vi "Add Item.vi"(6 "ForceAdd(F)":bool, 7 "Type":refnum<class "Generic.lvclass">, 8 "错误输入（无错误）":errorcluster, 9 "TypeGUID":string, 10 "Name":string, 11 "Section in":refnum<data-value>) -> (0 "错误输出":errorcluster, 2 "Item":refnum<data-value>, 3 "Section out":refnum<data-value>, 4 "Newly Created?":bool)   [LabVIEW 2013, in "Hierarchy Framework.lvlib" / "Section.lvclass"]
uses:
  Section.lvclass
  Item/Item.lvclass
  Generic/Generic.lvclass
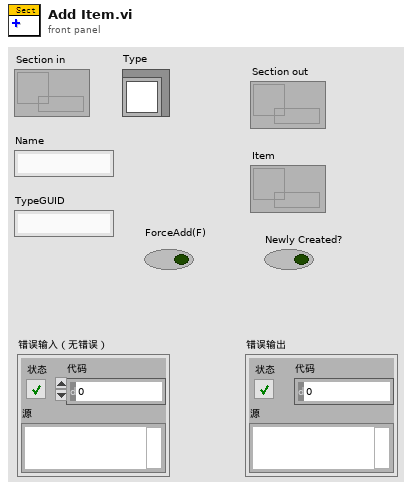
[diagram p1: front panel]
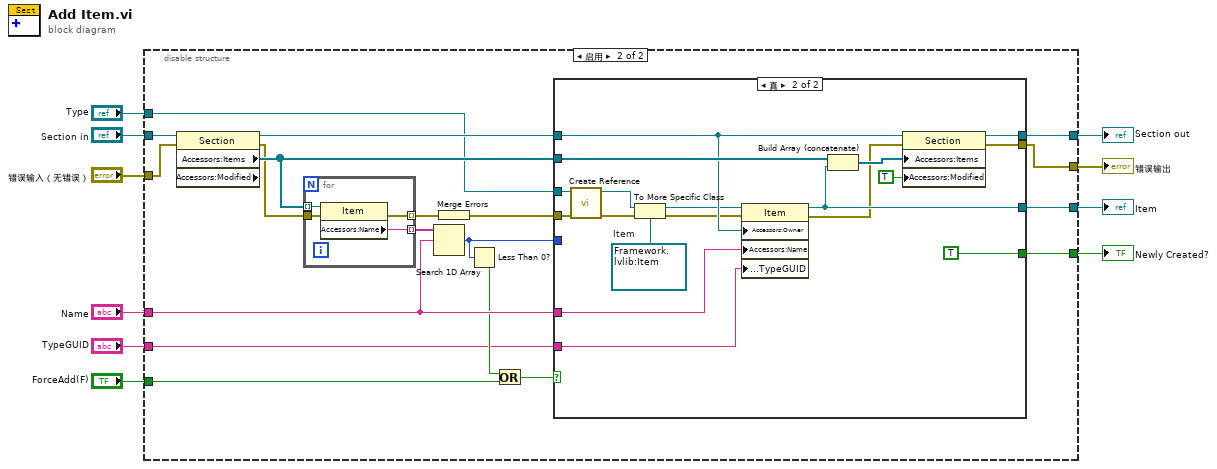
[diagram p0: block diagram]
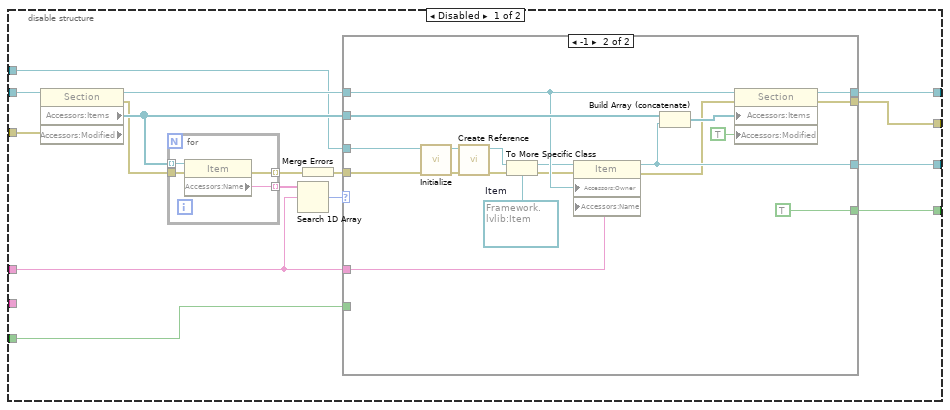
[diagram p2: hidden frame]
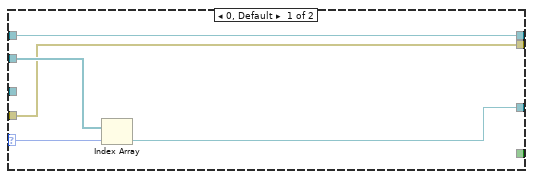
[diagram p3: hidden frame]
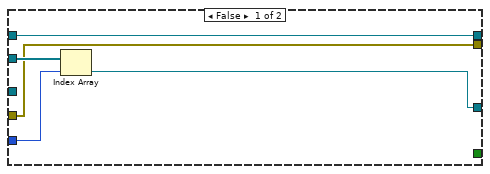
[diagram p4: hidden frame]
diagram:
  n1 = disable-structure shown="启用" {
    disable-tunnel: [w25 w72] -> w10
    disable-tunnel: [w24 w71] -> w9
    disable-tunnel: "Section in" -> [w23 w70]
    disable-tunnel: "错误输入（无错误）" -> [w22 w69]
    disable-tunnel: [w21 w68] -> w6
    disable-tunnel: "Name" -> [w20 w67]
    disable-tunnel: [w13 w61] -> w4
    disable-tunnel: "ForceAdd(F)" -> [w12 w58]
    disable-tunnel: "Type" -> [w11 w60]
    disable-tunnel: "TypeGUID" -> [_ w55]
    frame Disabled {
      n2 = property class="Section" props=["Accessors:Items", "Accessors:Modified"](reference=w23, error in=w22) -> (reference out=w19:refnum<data-value>, error out=w15:errorcluster, "Accessors:Items"=w26:refnum<data-value>[])  [unwired: 1 out]
      n3 = for {
        tunnel: w26 -> [w54] mode=indexing
        tunnel: [w53] -> w14 mode=indexing
        tunnel: w15 -> [w52]
        tunnel: [w51] -> w16 mode=indexing
        n4 = property class="Item"(reference=w54, error in=w52) -> (error out=w51:errorcluster, "Accessors:Name"=w53:string)  [unwired: 1 out]
      }
      n5 = Search 1D Array(1D array=w14, element=w20) -> (index of element=w17:i32)  [unwired: 1 in]
      n6 = Merge Errors(w16) -> (w18:errorcluster)
      n7 = case shown="-1" w17 {
        selector: w17 -> [w30 _]
        tunnel: w18 -> [w28 w37]
        tunnel: w19 -> [w27 w46]
        tunnel: w26 -> [w31 w50]
        tunnel: w20 -> [_ w39]
        tunnel: [w29 w41] -> w24
        tunnel: [w28 w48] -> w25
        tunnel: [_ TRUE] -> w21
        tunnel: [w27 w34] -> w13
        tunnel: w12 -> [_ _]
        tunnel: w11 -> [_ w32]
        frame 0, Default {
          n8 = Index Array(array=w31, index=w30) -> (element=w29:refnum<data-value>)
        }
        frame -1 {
          w33 = refnum<data-value> refnum  # Item
          n9 = call-dynamic "Initialize.vi"("error in (no error)"=w37, "Generic输入"=w32) -> ("error out"=w35:errorcluster, "Generic输出"=w36:refnum<class "Generic.lvclass">)  [unwired: 8 in]
          n10 = call "Create Reference.vi"("error in (no error)"=w35, "Generic"=w36) -> ("error out"=w44:errorcluster, "Generic Reference"=w45:refnum<data-value>)  [unwired: 8 in]
          n11 = To More Specific Class(target class=w33, reference=w45, error in=w44) -> (specific class reference=w42:refnum<data-value>, error out=w43:errorcluster)
          n12 = property class="Item"(reference=w42, error in=w43, "Accessors:Owner"=w46, "Accessors:Name"=w39) -> (reference out=w41:refnum<data-value>, error out=w40:errorcluster)
          n13 = Build Array (concatenate)(w50, w41) -> (w49:refnum<data-value>[])
          n14 = property class="Section"(reference=w46, error in=w40, "Accessors:Items"=w49, "Accessors:Modified"=TRUE ("Modified")) -> (reference out=w34:refnum<data-value>, error out=w48:errorcluster)
        }
      }
    }
    frame Enabled {
      n15 = property class="Section" props=["Accessors:Items", "Accessors:Modified"](reference=w70, error in=w69) -> (reference out=w66:refnum<data-value>, error out=w63:errorcluster, "Accessors:Items"=w73:refnum<data-value>[])  [unwired: 1 out]
      n16 = for {
        tunnel: w73 -> [w100] mode=indexing
        tunnel: [w99] -> w62 mode=indexing
        tunnel: w63 -> [w98]
        tunnel: [w97] -> w64 mode=indexing
        n17 = property class="Item"(reference=w100, error in=w98) -> (error out=w97:errorcluster, "Accessors:Name"=w99:string)  [unwired: 1 out]
      }
      n18 = Search 1D Array(1D array=w62, element=w67) -> (index of element=w56:i32)  [unwired: 1 in]
      n19 = Merge Errors(w64) -> (w65:errorcluster)
      n20 = Less Than 0?(x=w56) -> (x < 0?=w59:bool)
      n21 = Or(x=w59, y=w58) -> (x .or. y?=w57:bool)
      n22 = case shown="真" w57 {
        tunnel: w65 -> [w76 w83]
        tunnel: w66 -> [w75 w92]
        tunnel: w73 -> [w78 w96]
        tunnel: w67 -> [_ w85]
        tunnel: [w77 w87] -> w71
        tunnel: [w76 w94] -> w72
        tunnel: [_ TRUE] -> w68
        tunnel: [w75 w82] -> w61
        tunnel: w60 -> [_ w80]
        tunnel: w56 -> [w74 _]
        tunnel: w55 -> [_ w79]
        frame False {
          n23 = Index Array(array=w78, index=w74) -> (element=w77:refnum<data-value>)
        }
        frame True {
          w81 = refnum<data-value> refnum  # Item
          n24 = call "Create Reference.vi"("error in (no error)"=w83, "Generic"=w80) -> ("error out"=w90:errorcluster, "Generic Reference"=w91:refnum<data-value>)  [unwired: 8 in]
          n25 = To More Specific Class(target class=w81, reference=w91, error in=w90) -> (specific class reference=w88:refnum<data-value>, error out=w89:errorcluster)
          n26 = property class="Item"(reference=w88, error in=w89, "Accessors:Owner"=w92, "Accessors:Name"=w85, "Accessors:TypeGUID"=w79) -> (reference out=w87:refnum<data-value>, error out=w86:errorcluster)
          n27 = Build Array (concatenate)(w96, w87) -> (w95:refnum<data-value>[])
          n28 = property class="Section"(reference=w92, error in=w86, "Accessors:Items"=w95, "Accessors:Modified"=TRUE ("Modified")) -> (reference out=w82:refnum<data-value>, error out=w94:errorcluster)
        }
      }
    }
  }
  "错误输出" <- w10
  "Item" <- w9
  "Newly Created?" <- w6
  "Section out" <- w4
